vi "example 8 - mouse click.vi"() -> ()   [LabVIEW 2020]
uses:
  ui-testing/ui-testing.lvlib
panel:
  in  "n-label-unvis":bool
  in  "n-label-vis":bool
  in  "m-label-unvis":bool
  in  "m-label-vis":bool
  out "String":string
  in  "Reset":bool
  in  "Hide toolbar":bool
  in  "Show toolbar":bool
  in  "Hide menu":bool
  in  "Show menu":bool
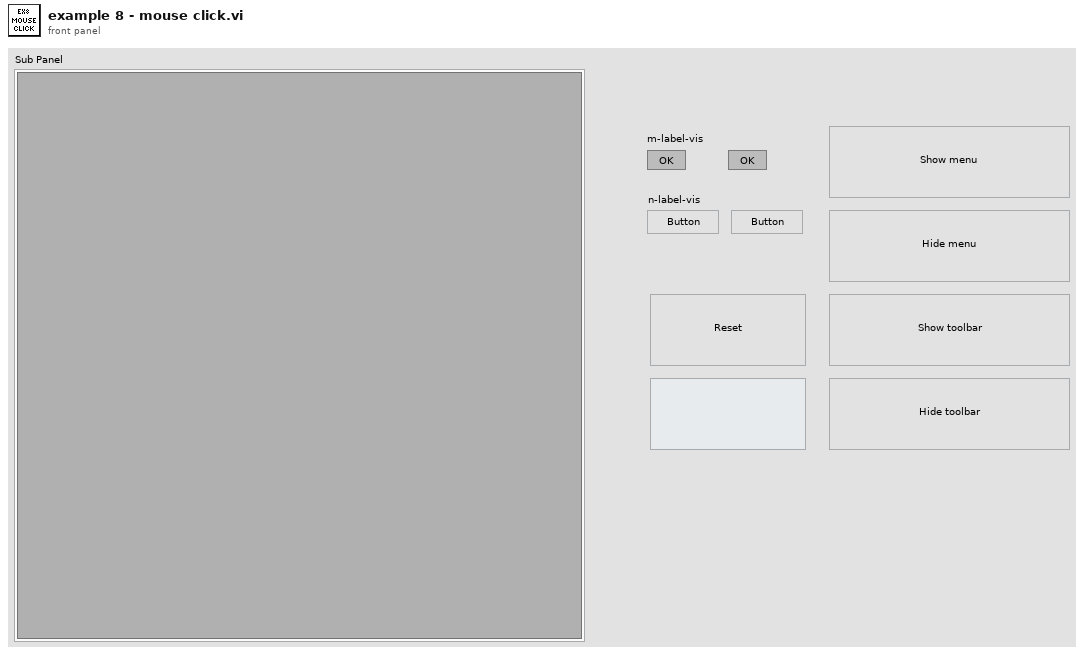
[diagram p1: front panel]
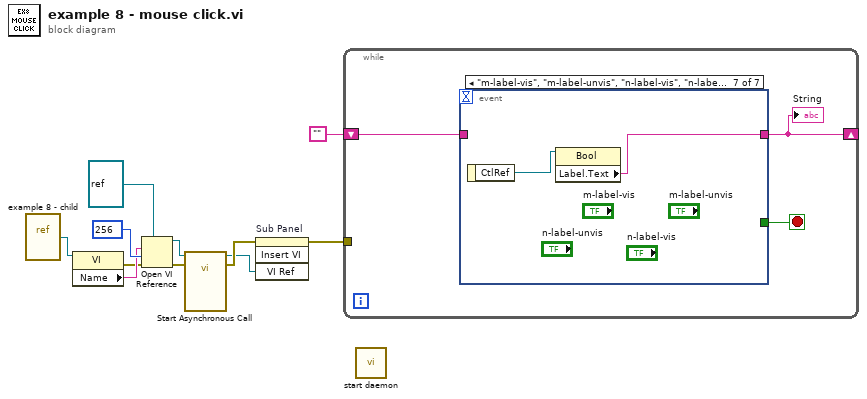
[diagram p0: block diagram]
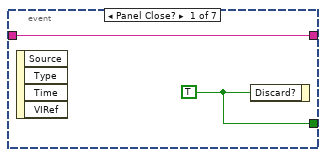
[diagram p2: hidden frame]
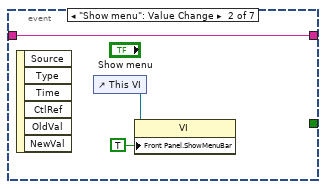
[diagram p3: hidden frame]
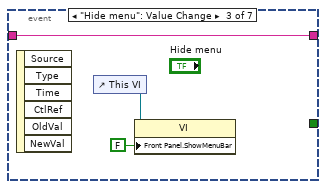
[diagram p4: hidden frame]
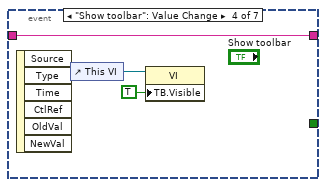
[diagram p5: hidden frame]
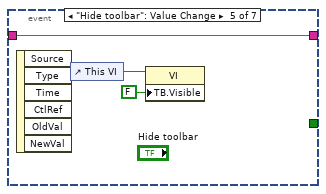
[diagram p6: hidden frame]
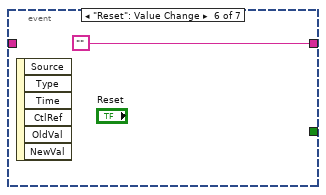
[diagram p7: hidden frame]
diagram:
  n1 = vi-ref "example 8 - child.vi"() -> (w7:refnum<vi>)
  n2 = property class="VI"(reference=w7) -> (error out=w5:errorcluster, "Name"=w6:string)  [unwired: 1 in, 1 out]
  n3 = Open VI Reference(type specifier VI Refnum (for type only)=refnum<vi> refnum, vi path=w6, options=256 ("call and forget"), error in (no error)=w5) -> (vi reference=w9:refnum<vi>, error out=w8:errorcluster)  [unwired: 2 in]
  n4 = call-by-ref "Start Asynchronous Call"(reference=w9, error in=w8) -> (reference out=w3:refnum<vi>, error out=w4:errorcluster)  [unwired: 12 in]
  n5 = invoke on="Sub Panel" class="SubPnl" method="Insert VI"(error in=w4, "VI Ref"=w3) -> (error out=w1:errorcluster)  [unwired: 2 in, 3 out]
  n6 = while {
    shift-right: [w12] -> _
    shift-left: "" -> [w13]
    tunnel: w1 -> [_]
    stop <- w14 stop-if-true
    n7 = event shown="[6] \"m-label-vis\", \"m-label-unvis\", \"n-label-vis\", \"n-label-unvis\": Value Change" {
      selector: _ -> [_ _ _ _ _ _ _]
      dyn-events: _ -> [_ _ _ _ _ _ _]
      timeout: _ -> [_ _ _ _ _ _ _]
      tunnel: [w16 _ _ _ _ _ _] -> w14
      tunnel: [w15 w17 w20 w23 w26 "" w30] -> w12
      tunnel: w13 -> [w15 w17 w20 w23 w26 _ _]
      event Panel Close? {
        w16 = TRUE
        n8 = event-data() -> ()  [unwired: 1 in, 4 out]
        n9 = event-data("Discard?"=w16) -> ()  [unwired: 1 in, 1 out]
      }
      event "Show menu": Value Change {
        n10 = event-data() -> ()  [unwired: 1 in, 6 out]
        n11 = control-ref of="This VI"() -> (w19:refnum<vi>)
        n12 = property class="VI"(reference=w19, "Front Panel.ShowMenuBar"=TRUE ("Front Panel Window:Show Menu Bar")) -> ()  [unwired: 1 in, 2 out]
      }
      event "Hide menu": Value Change {
        n13 = event-data() -> ()  [unwired: 1 in, 6 out]
        n14 = control-ref of="This VI"() -> (w22:refnum<vi>)
        n15 = property class="VI"(reference=w22, "Front Panel.ShowMenuBar"=FALSE ("Front Panel Window:Show Menu Bar")) -> ()  [unwired: 1 in, 2 out]
      }
      event "Show toolbar": Value Change {
        n16 = event-data() -> ()  [unwired: 1 in, 6 out]
        n17 = control-ref of="This VI"() -> (w25:refnum<vi>)
        n18 = property class="VI"(reference=w25, "TB.Visible"=TRUE ("Tool Bar:Visible")) -> ()  [unwired: 1 in, 2 out]
      }
      event "Hide toolbar": Value Change {
        n19 = event-data() -> ()  [unwired: 1 in, 6 out]
        n20 = control-ref of="This VI"() -> (w28:refnum<vi>)
        n21 = property class="VI"(reference=w28, "TB.Visible"=FALSE ("Tool Bar:Visible")) -> ()  [unwired: 1 in, 2 out]
      }
      event "Reset": Value Change {
        n22 = event-data() -> ()  [unwired: 1 in, 6 out]
      }
      event "m-label-vis", "m-label-unvis", "n-label-vis", "n-label-unvis": Value Change {
        n23 = event-data() -> ("CtlRef"=w31:refnum<vi>)  [unwired: 1 in]
        n24 = property class="Bool"(reference=w31) -> ("Label.Text"=w30:string)  [unwired: 1 in, 2 out]
      }
    }
    "String" <- w12
  }
  n25 = call "start daemon.vi"() -> ()  [unwired: 11 in, 1 out]
